vi "Set image name.vi"(8 "error in (no error)":errorcluster) -> (0 "error out":errorcluster, 3 "image name":string)   [LabVIEW 2016]
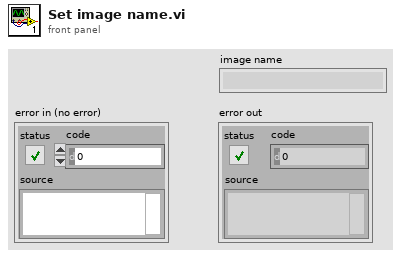
[diagram p1: front panel]
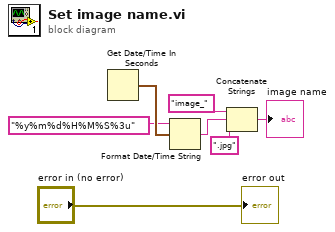
[diagram p0: block diagram]
diagram:
  n1 = Get Date/Time In Seconds() -> (seconds since 1Jan1904=w4:timestamp)
  n2 = Format Date/Time String(time format string (%c)="%y%m%d%H%M%S%3u", seconds (now)=w4) -> (date/time string=w7:string)  [unwired: 1 in]
  n3 = Concatenate Strings("image_" ("string"), w7, ".jpg" ("string")) -> (→"image name":string)
  "error out" <- "error in (no error)"
